vi "Create Topic Array.vi"(10 "IoT Parameters":T2={"MQTT Broker"={"address (IP)"="azwqv45vu9vjz.iot.us-east-2.amazonaws.com", "port"=8883}, "cert path"={"client cert file"=path "C:/Users/Jembedded/Downloads/aa6df4a004-certificate.pem.crt", "client key file"=path "C:/Users/Jembedded/Downloads/aa6df4a004-private.pem.key"}, "Topic Prefix"="", "Serial Number"="", "Subscriptions"=[]}) -> (2 "Topic Array":cluster{"Topic":string, "QoS":T1}[](array[cluster]))   [LabVIEW 2018]
uses:
  Controls/IoT Parameters.ctl
  Controls/certs.ctl
  MQTT/Controls/QoS.ctl
  AWS_IoT.lvlib
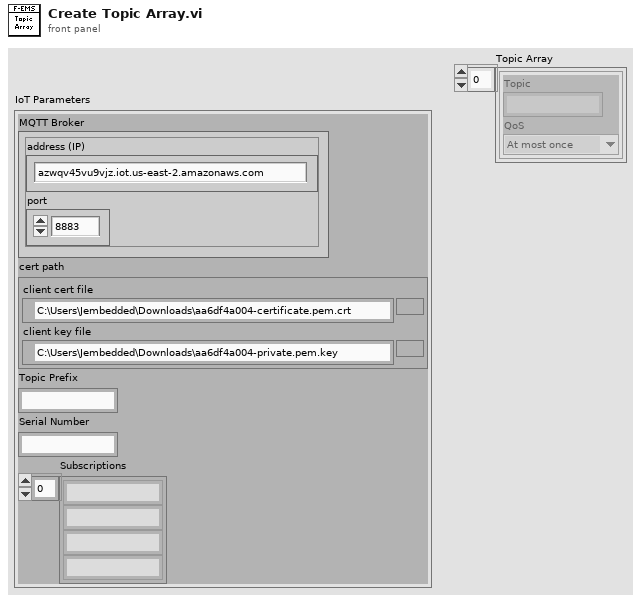
[diagram p1: front panel]
types:
  T1 = typedef "AWS_IoT.lvlib/QoS.ctl" = enum8{"At most once", "At least once", "Exactly once", "Reserved"}
  T2 = typedef "IoT Parameters.ctl" = cluster{"MQTT Broker":cluster{"address (IP)":string, "port":u16}, "cert path":T3, "Topic Prefix":string, "Serial Number":string, "Subscriptions":string[]}
  T3 = typedef "AWS_IoT.lvlib/certs.ctl" = cluster{"client cert file":path, "client key file":path}
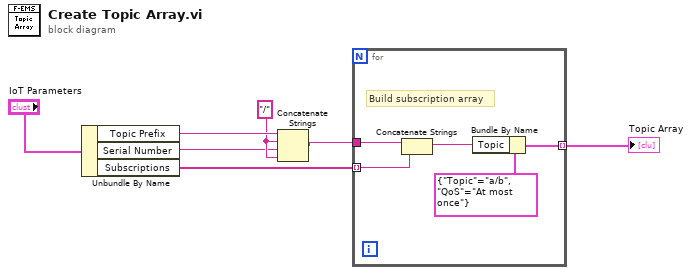
[diagram p0: block diagram]
diagram:
  w5 = "/" ("string")
  n1 = Unbundle By Name("IoT Parameters") -> ("Topic Prefix"=w6:string, "Serial Number"=w4:string, "Subscriptions"=w3:string[])
  n2 = Concatenate Strings(w6, w5, w4, w5) -> (w2:string)
  n3 = for {
    tunnel: w3 -> [w11] mode=indexing
    tunnel: w2 -> [w12]
    tunnel: [w8] -> w1 mode=indexing
    # "Build subscription array"
    n4 = Concatenate Strings(w12, w11) -> (w9:string)
    n5 = Bundle By Name(cluster=cluster{"Topic":string, "QoS":T1} {"Topic"="a/b", "QoS"=enum."At most once"} ("Subscription Info"), "Topic"=w9) -> (w8:cluster{"Topic":string, "QoS":T1})
  }
  "Topic Array" <- w1
